vi "LVJSON Dump.vi"(4 "PPIsValue? (F)":bool, 6 "PPIndent (0)":i32, 8 "error in (no error)":errorcluster, 10 "Pretty Print? (F)":bool, 11 "Root Element in":T1) -> (0 "error out":errorcluster, 2 "Key":string, 3 "JSON out":string)   [LabVIEW 2019, in "labview_json.lvlib"]
uses:
  labview_json.lvlib
  Element.ctl
  Element Type.ctl
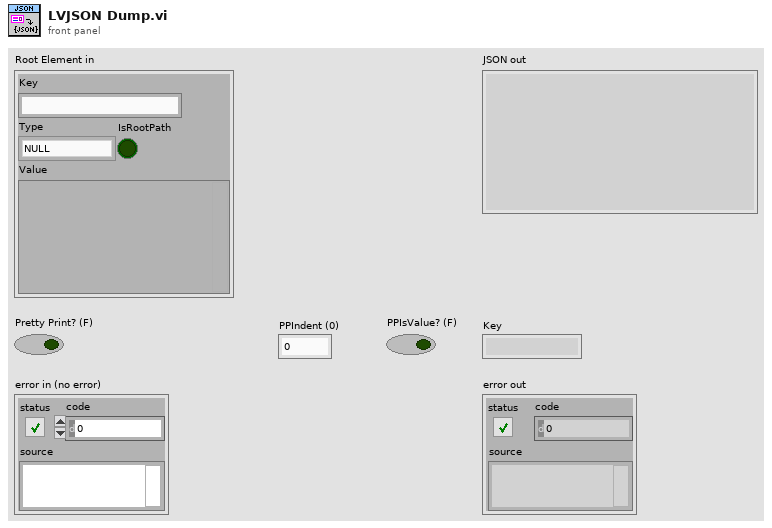
[diagram p1: front panel]
types:
  T1 = typedef "labview_json.lvlib/Element.ctl" = cluster{"Key":string, "Type":T2, "Value":variant, "IsRootPath":bool}
  T2 = typedef "labview_json.lvlib/Element Type.ctl" = enum8{"NULL", "OBJECT", "ARRAY", "BOOL", "INT", "UINT", "FLOAT", "STRING"}
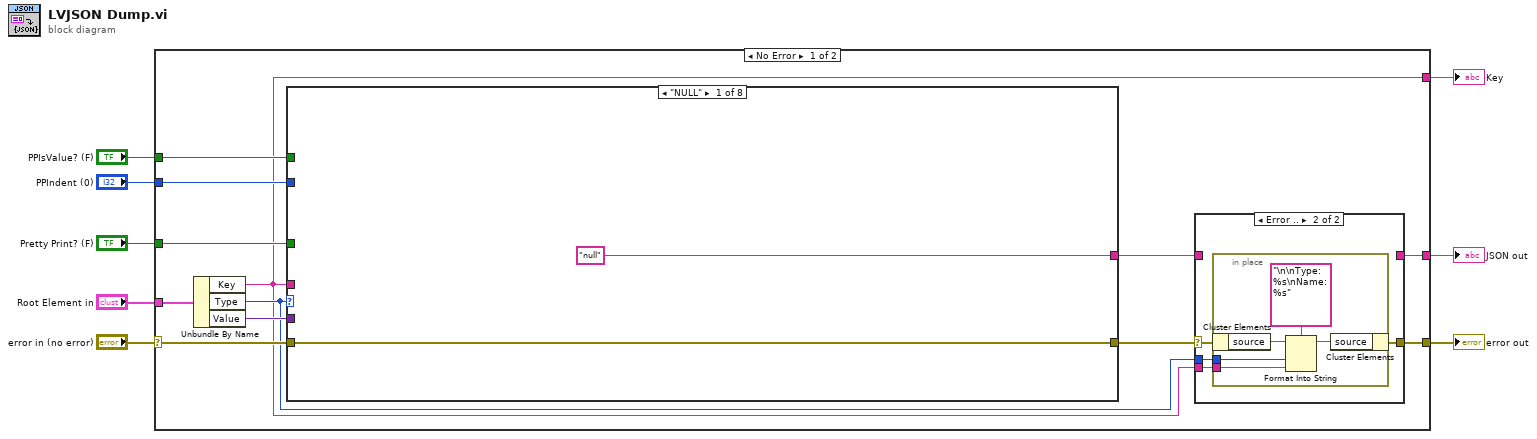
[diagram p0: block diagram]
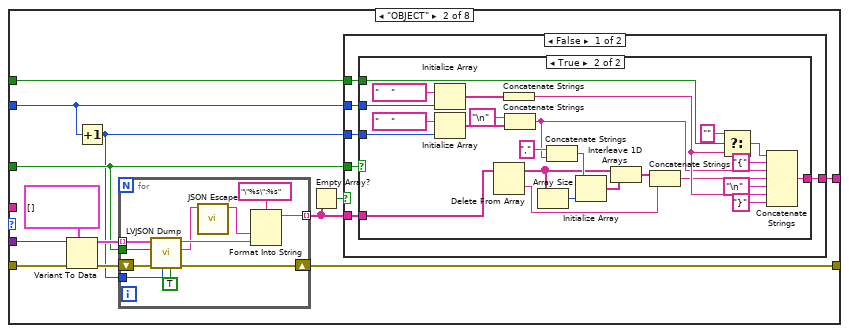
[diagram p3: hidden frame]
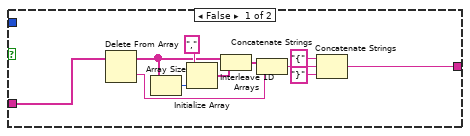
[diagram p4: hidden frame]
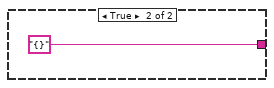
[diagram p5: hidden frame]
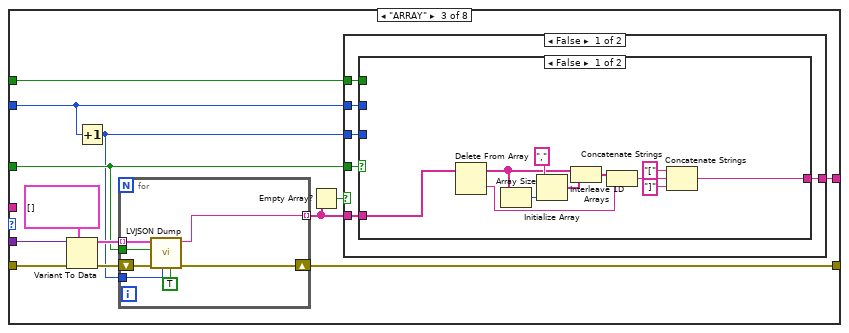
[diagram p6: hidden frame]
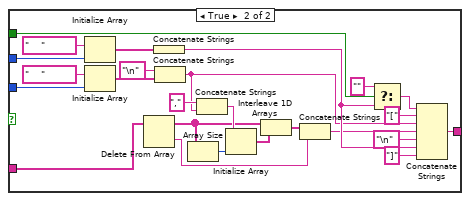
[diagram p7: hidden frame]
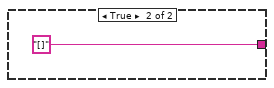
[diagram p8: hidden frame]
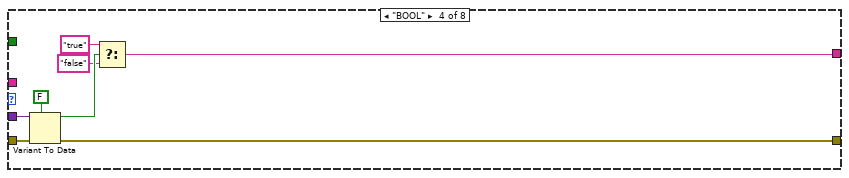
[diagram p9: hidden frame]
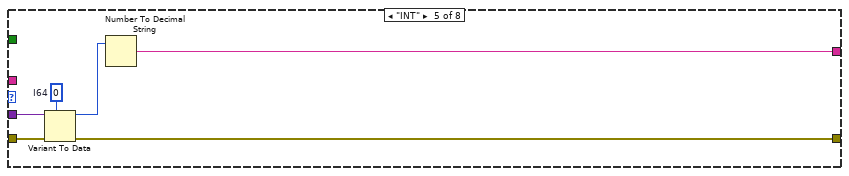
[diagram p10: hidden frame]
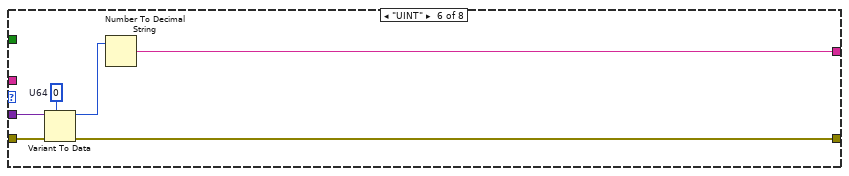
[diagram p11: hidden frame]
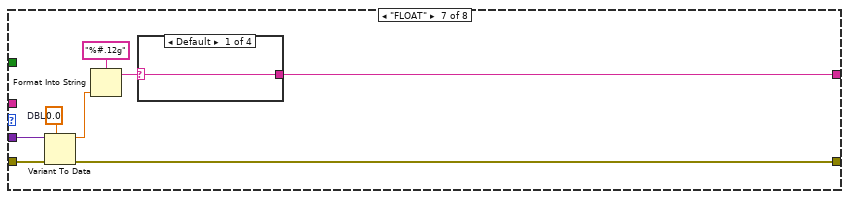
[diagram p12: hidden frame]
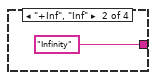
[diagram p13: hidden frame]
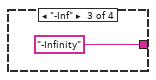
[diagram p14: hidden frame]
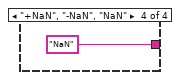
[diagram p15: hidden frame]
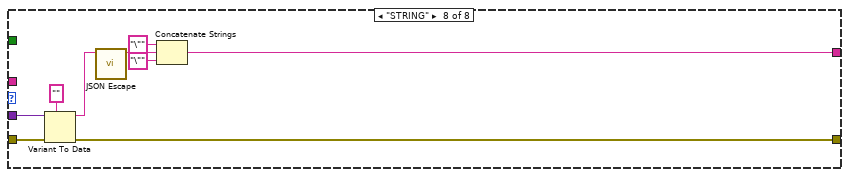
[diagram p16: hidden frame]
diagram:
  n1 = case shown="No Error" "error in (no error)" {
    selector: "error in (no error)" -> [w18 w205]
    tunnel: "Root Element in" -> [w20 _]
    tunnel: [w12 _] -> w7
    tunnel: [w11 w205] -> w5
    tunnel: [w10 _] -> w4
    tunnel: "Pretty Print? (F)" -> [w17 _]
    tunnel: "PPIndent (0)" -> [w16 _]
    tunnel: "PPIsValue? (F)" -> [w15 _]
    frame No Error {
      n2 = Unbundle By Name(w20) -> ("Key"=w12:string, "Type"=w13:T2, "Value"=w19:variant)
      n3 = case shown="\"NULL\"" w13 {
        tunnel: w19 -> [_ w46 w113 w169 w175 w181 w189 w202]
        tunnel: w12 -> [_ _ _ _ _ _ _ _]
        tunnel: w18 -> [w32 w44 w111 w171 w177 w183 w191 w204]
        tunnel: [w32 w42 w109 w170 w176 w182 w190 w203] -> w14
        tunnel: ["null" w40 w107 w164 w172 w178 w184 w198] -> w9
        tunnel: w17 -> [_ w39 w106 _ _ _ _ _]
        tunnel: w16 -> [_ w37 w104 _ _ _ _ _]
        tunnel: w15 -> [_ w38 w105 _ _ _ _ _]
        frame "NULL" {
        }
        frame "OBJECT" {
          n4 = Variant To Data(error in=w44, type=T1[] [], Variant=w46) -> (data=w41:T1[], error out=w43:errorcluster)
          n5 = Increment(x=w37) -> (x+1=w36:i32)
          n6 = for {
            tunnel: w41 -> [w98] mode=indexing
            shift-right: [w99] -> w42
            shift-left: w43 -> [w100]
            tunnel: [w96] -> w35 mode=indexing
            tunnel: w39 -> [w92]
            tunnel: w36 -> [w91]
            n7 = call "LVJSON Dump.vi"("PPIsValue? (F)"=TRUE ("Pretty Print Is Value? (F)"), "PPIndent (0)"=w91, "error in (no error)"=w100, "Pretty Print? (F)"=w92, "Root Element in"=w98) -> ("error out"=w99:errorcluster, "Key"=w94:string, "JSON out"=w97:string)  [unwired: 4 in]
            n8 = call "JSON Escape.vi"("String"=w94) -> ("Escaped String"=w93:string)  [unwired: 9 in, 1 out]
            n9 = Format Into String(format string="\"%s\":%s", w93, w97) -> (resulting string=w96:string)  [unwired: 2 in, 1 out]
          }
          n10 = Empty Array?(array=w35) -> (empty?=w34:bool)
          n11 = case shown="False" w34 {
            tunnel: [w52 "{}"] -> w40
            tunnel: w39 -> [w51 _]
            tunnel: w38 -> [w50 _]
            tunnel: w37 -> [w49 _]
            tunnel: w36 -> [w48 _]
            tunnel: w35 -> [w47 _]
            frame False {
              n12 = case shown="True" w51 {
                tunnel: w47 -> [w63 w69]
                tunnel: [w59 w65] -> w52
                tunnel: w50 -> [_ w67]
                tunnel: w49 -> [_ w68]
                tunnel: w48 -> [_ w66]
                frame False {
                  n13 = Delete From Array(array=w63) -> (deleted portion=w53:string, array with subset deleted=w56:string[])  [unwired: 2 in]
                  n14 = Array Size(array=w56) -> (size(s)=w58:i32)
                  n15 = Initialize Array(",", w58) -> (w55:string[])
                  n16 = Interleave 1D Arrays(w56, w55) -> (w54:string[])
                  n17 = Concatenate Strings(w54, w53) -> (w60:string)
                  n18 = Concatenate Strings("{" ("string"), w60, "}" ("string")) -> (w59:string)
                }
                frame True {
                  n19 = Initialize Array("    " ("element"), w68) -> (w86:string[])
                  n20 = Initialize Array("    " ("element"), w66) -> (w82:string[])
                  n21 = Delete From Array(array=w69) -> (deleted portion=w84:string, array with subset deleted=w79:string[])  [unwired: 2 in]
                  n22 = Concatenate Strings(w86) -> (w88:string)
                  n23 = Concatenate Strings("\n" ("element"), w82) -> (w64:string)
                  n24 = Array Size(array=w79) -> (size(s)=w78:i32)
                  n25 = Concatenate Strings("," ("string"), w64) -> (w85:string)
                  n26 = Initialize Array(w85, w78) -> (w80:string[])
                  n27 = Interleave 1D Arrays(w79, w80) -> (w81:string[])
                  n28 = Concatenate Strings(w81, w84) -> (w83:string)
                  n29 = Select(t="", s=w67, f=w88) -> (s? t:f=w87:string)
                  n30 = Concatenate Strings(w87, "{" ("string"), w64, w83, "\n" ("element"), w88, "}" ("string")) -> (w65:string)
                }
              }
            }
            frame True {
            }
          }
        }
        frame "ARRAY" {
          n31 = Variant To Data(error in=w111, type=T1[] [], Variant=w113) -> (data=w108:T1[], error out=w110:errorcluster)
          n32 = Increment(x=w104) -> (x+1=w103:i32)
          n33 = for {
            tunnel: w108 -> [w161] mode=indexing
            shift-right: [w162] -> w109
            shift-left: w110 -> [w163]
            tunnel: [w157] -> w102 mode=indexing
            tunnel: w106 -> [w160]
            tunnel: w103 -> [w159]
            n34 = call "LVJSON Dump.vi"("PPIsValue? (F)"=TRUE ("Pretty Print Is Value? (F)"), "PPIndent (0)"=w159, "error in (no error)"=w163, "Pretty Print? (F)"=w160, "Root Element in"=w161) -> ("error out"=w162:errorcluster, "JSON out"=w157:string)  [unwired: 4 in, 1 out]
          }
          n35 = Empty Array?(array=w102) -> (empty?=w101:bool)
          n36 = case shown="False" w101 {
            tunnel: [w119 "[]"] -> w107
            tunnel: w106 -> [w118 _]
            tunnel: w105 -> [w117 _]
            tunnel: w104 -> [w116 _]
            tunnel: w103 -> [w115 _]
            tunnel: w102 -> [w114 _]
            frame False {
              n37 = case shown="False" w118 {
                tunnel: w114 -> [w130 w136]
                tunnel: [w126 w132] -> w119
                tunnel: w117 -> [_ w134]
                tunnel: w116 -> [_ w135]
                tunnel: w115 -> [_ w133]
                frame False {
                  n38 = Delete From Array(array=w130) -> (deleted portion=w120:string, array with subset deleted=w123:string[])  [unwired: 2 in]
                  n39 = Array Size(array=w123) -> (size(s)=w125:i32)
                  n40 = Initialize Array(",", w125) -> (w122:string[])
                  n41 = Interleave 1D Arrays(w123, w122) -> (w121:string[])
                  n42 = Concatenate Strings(w121, w120) -> (w127:string)
                  n43 = Concatenate Strings("[" ("string"), w127, "]" ("string")) -> (w126:string)
                }
                frame True {
                  n44 = Initialize Array("    " ("element"), w135) -> (w153:string[])
                  n45 = Initialize Array("    " ("element"), w133) -> (w149:string[])
                  n46 = Delete From Array(array=w136) -> (deleted portion=w151:string, array with subset deleted=w146:string[])  [unwired: 2 in]
                  n47 = Concatenate Strings(w153) -> (w155:string)
                  n48 = Concatenate Strings("\n" ("element"), w149) -> (w131:string)
                  n49 = Array Size(array=w146) -> (size(s)=w145:i32)
                  n50 = Concatenate Strings("," ("string"), w131) -> (w152:string)
                  n51 = Initialize Array(w152, w145) -> (w147:string[])
                  n52 = Interleave 1D Arrays(w146, w147) -> (w148:string[])
                  n53 = Concatenate Strings(w148, w151) -> (w150:string)
                  n54 = Select(t="", s=w134, f=w155) -> (s? t:f=w154:string)
                  n55 = Concatenate Strings(w154, "[" ("string"), w131, w150, "\n" ("element"), w155, "]" ("string")) -> (w132:string)
                }
              }
            }
            frame True {
            }
          }
        }
        frame "BOOL" {
          n56 = Variant To Data(error in=w171, type=FALSE, Variant=w169) -> (data=w167:bool, error out=w170:errorcluster)
          n57 = Select(t="true", s=w167, f="false") -> (s? t:f=w164:string)
        }
        frame "INT" {
          w174 = i64 0  # I64
          n58 = Variant To Data(error in=w177, type=w174, Variant=w175) -> (data=w173:i64, error out=w176:errorcluster)
          n59 = Number To Decimal String(number=w173) -> (decimal integer string=w172:string)  [unwired: 1 in]
        }
        frame "UINT" {
          w180 = u64 0  # U64
          n60 = Variant To Data(error in=w183, type=w180, Variant=w181) -> (data=w179:u64, error out=w182:errorcluster)
          n61 = Number To Decimal String(number=w179) -> (decimal integer string=w178:string)  [unwired: 1 in]
        }
        frame "FLOAT" {
          w188 = 0.0  # DBL
          n62 = Variant To Data(error in=w191, type=w188, Variant=w189) -> (data=w187:dbl, error out=w190:errorcluster)
          n63 = Format Into String(format string="%#.12g", w187) -> (resulting string=w185:string)  [unwired: 2 in, 1 out]
          n64 = case shown="Default" w185 {
            selector: w185 -> [w192 _ _ _]
            tunnel: [w192 "Infinity" "-Infinity" "NaN"] -> w184
            frame Default {
            }
            frame "+Inf", "Inf" {
            }
            frame "-Inf" {
            }
            frame "+NaN", "-NaN", "NaN" {
            }
          }
        }
        frame "STRING" {
          n65 = Variant To Data(error in=w204, type="", Variant=w202) -> (data=w200:string, error out=w203:errorcluster)
          n66 = call "JSON Escape.vi"("String"=w200) -> ("Escaped String"=w199:string)  [unwired: 9 in, 1 out]
          n67 = Concatenate Strings("\"" ("string"), w199, "\"" ("string")) -> (w198:string)
        }
      }
      n68 = case shown="Error .." w14 {
        selector: w14 -> [w22 w26]
        tunnel: [w22 w25] -> w11
        tunnel: w13 -> [_ w24]
        tunnel: w12 -> [_ w23]
        tunnel: [w21 _] -> w10
        tunnel: w9 -> [w21 _]
        frame No Error {
        }
        frame Error {
          n69 = in-place {
            in-place-border: w24 -> [w28]
            in-place-border: w23 -> [w27]
            n70 = in-place-cluster #1(w26) -> ("source"=w31:string)
            n71 = Format Into String(format string="\n\nType: %s\nName: %s", initial string=w31, w28, w27) -> (resulting string=w30:string)  [unwired: 1 in, 1 out]
            n72 = in-place-cluster #1("source"=w30) -> (w25:errorcluster)
          }
        }
      }
    }
    frame Error {
    }
  }
  "JSON out" <- w4
  "error out" <- w5
  "Key" <- w7
